vi "ImageRecon.vi"(7 "Logging queue element in":T1={"Imaging Protocol"=enum."Live Imaging", "Number of Trials"=0, "Frame Size"=512, "# Averaged frames"=0, "Dwell time (us)"=0.0, "Index of Z-plane"=0, "Timelapse?"=FALSE, "Logging process is active"=FALSE, "Speed logging enabled"=FALSE, "tdms file ref"=refnum, "path"=path "", "Trial Number"=0, "Expected # points acquired"=FALSE, "Manually stopped"=FALSE, "Last trial"=FALSE, "Ch0 data"=[], "Ch1 data"=[], "Image Time"=[], "Continuous Time"=[], "Points acquired"={"Ch0 last trial"=0, "Ch1 last trial"=0, "All trials"=0}, "HW Timings File"=refnum} {"Frame Size" items=["100X100"=100, "128X128"=128, "200X200"=200, "256X256"=256, "512X512"=512, "1024x1024"=1024, "2048x2048"=2048]; "Dwell time (us)" format="%#.6g"}, 8 "Error In":errorcluster, 9 "Data":T5, 10 "Frame Size":T3=200 items=["100X100"=100, "128X128"=128, "200X200"=200, "256X256"=256, "512X512"=512, "1024x1024"=1024, "2048x2048"=2048], 11 "Image Array (in)":T6) -> (0 "Error Out":errorcluster, 1 "Ch1-Green":i16[][](graph), 2 "Ch0-Red":i16[][](graph), 3 "Image Array(out)":T6)   [LabVIEW 2017]
uses:
  Typedefs/Frame Size.ctl
  Queue/Live graphs queue/Typedefs/Live imaging queue element.ctl
  <vilib>/vision/Image Controls.llb/IMAQ Image.ctl
  Typedefs/Frame data dual cluster.ctl
  Typedefs/Logging queue element.ctl
  Typedefs/Imaging Protocols enum.ctl
  Typedefs/Acquired points count.ctl
  Global Variables/gl_Images.vi
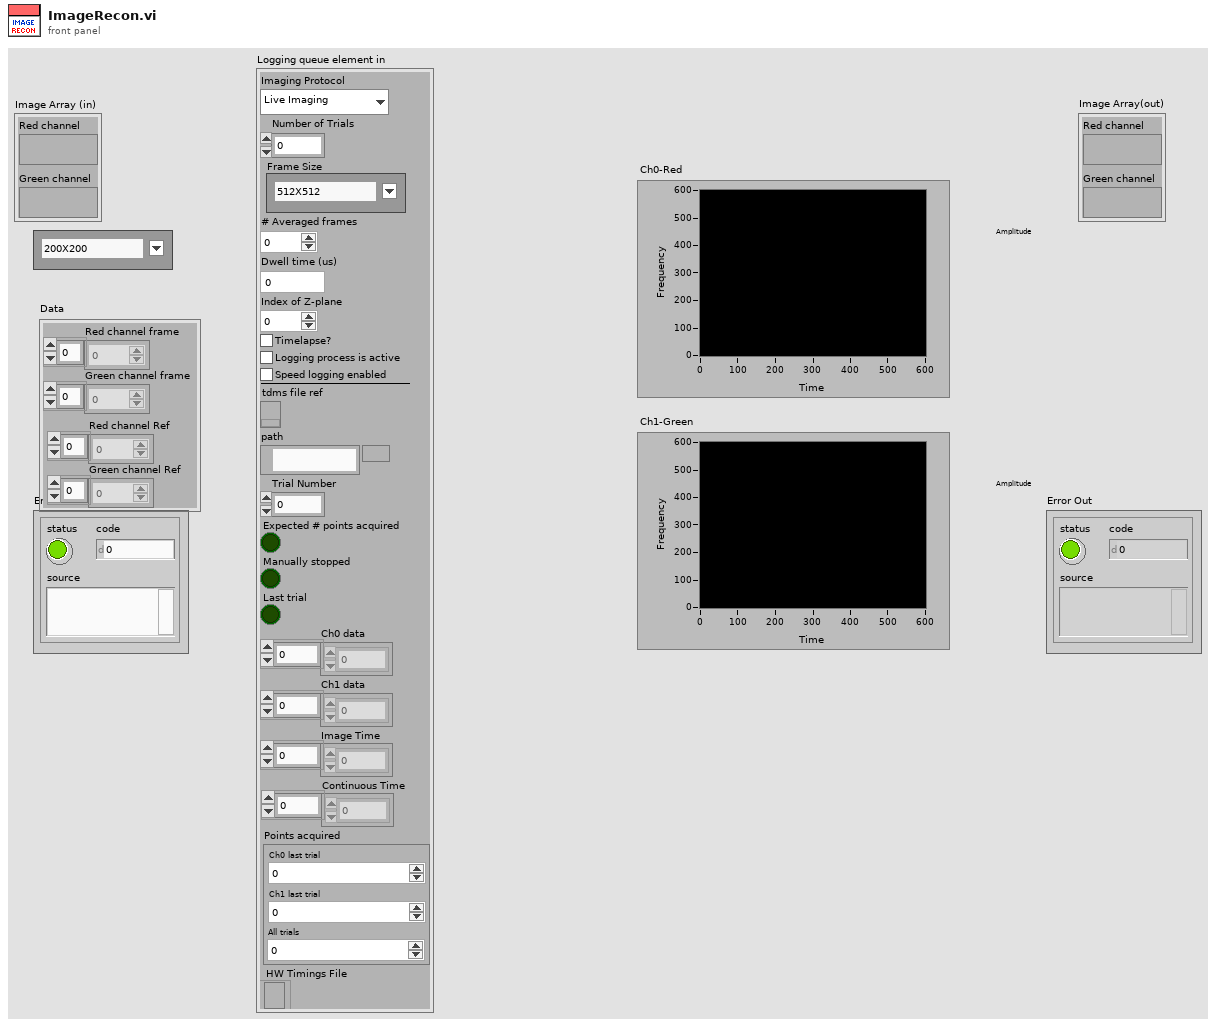
[diagram p1: front panel]
types:
  T1 = typedef "Logging queue element.ctl" = cluster{"Imaging Protocol":T2, "Number of Trials":u16, "Frame Size":T3, "# Averaged frames":u16, "Dwell time (us)":dbl, "Index of Z-plane":i32, "Timelapse?":bool, "Logging process is active":bool, "Speed logging enabled":bool, "tdms file ref":refnum<k34>, "path":path, "Trial Number":i32, "Expected # points acquired":bool, "Manually stopped":bool, "Last trial":bool, "Ch0 data":u32[], "Ch1 data":u32[], "Image Time":u64[], "Continuous Time":u64[], "Points acquired":T4, "HW Timings File":refnum<file>}
  T2 = typedef "Imaging Protocols enum.ctl" = enum16{"AOL Z-Stack", "Motor Z Stack", "Functional Acquisition", "Single Plane Acquisition", "Volume Acquisition", "Live Imaging", "Live Plane Imaging", "Live Volume Imaging"}
  T3 = typedef "Frame Size.ctl" = u16
  T4 = typedef "Acquired points count.ctl" = cluster{"Ch0 last trial":u64, "Ch1 last trial":u64, "All trials":u64}
  T5 = typedef "Frame data dual cluster.ctl" = cluster{"Red channel frame":dbl[], "Green channel frame":dbl[], "Red channel Ref":dbl[], "Green channel Ref":dbl[]}
  T6 = typedef "Live imaging queue element.ctl" = cluster{"Red channel":T7, "Green channel":T7}
  T7 = typedef "IMAQ Image.ctl" = refnum<image>
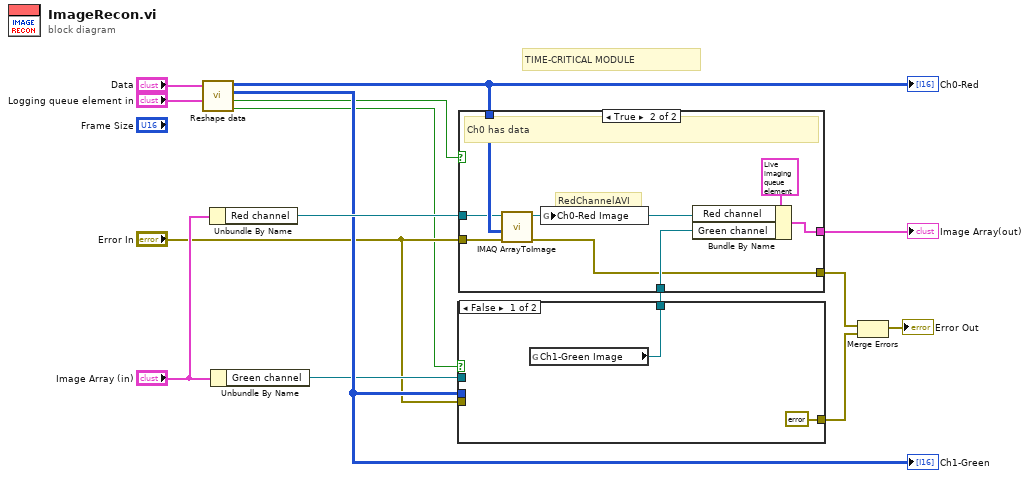
[diagram p0: block diagram]
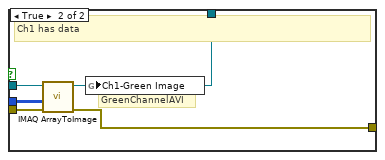
[diagram p2: hidden frame]
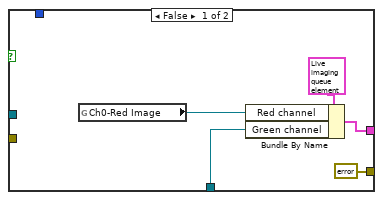
[diagram p3: hidden frame]
diagram:
  # "TIME-CRITICAL MODULE"
  n1 = call "Reshape data.vi"("Logging queue element in"="Logging queue element in", "Data"="Data") -> ("Ch1 has data"=w4:bool, "Ch0 has data"=w5:bool, "Ch1-Green"=w11:i16[][], "Ch0-Red"=w15:i16[][])  [unwired: 6 in]
  "Ch0-Red" <- w15
  "Ch1-Green" <- w11
  n2 = Unbundle By Name("Image Array (in)") -> ("Red channel"=w14:T7)
  n3 = Unbundle By Name("Image Array (in)") -> ("Green channel"=w10:T7)
  n4 = case shown="False" w4 {
    tunnel: w11 -> [_ w22]
    tunnel: w10 -> [_ w21]
    tunnel: "Error In" -> [_ w20]
    tunnel: [w17 w19] -> w6
    tunnel: [errorcluster {"status"=FALSE, "code"=0, "source"=""} ("error out") w18] -> w3
    frame False {
      n5 = global read "gl_Images.vi" "Ch1-Green Image"() -> (w17:T7)
    }
    frame True {
      # "GreenChannelAVI"
      # "Ch1 has data"
      n6 = call "IMAQ ArrayToImage"("error in (no error)"=w20, "Image Pixels (I16)"=w22, "Image"=w21) -> ("error out"=w18:errorcluster, "Image Out"=w19:T7)  [unwired: 7 in]
      n7 = global write "gl_Images.vi" "Ch1-Green Image"(w19) -> ()
    }
  }
  n8 = case shown="True" w5 {
    tunnel: w15 -> [_ w35]
    tunnel: w14 -> [_ w34]
    tunnel: [w25 w33] -> w13
    tunnel: "Error In" -> [_ w32]
    tunnel: w6 -> [w24 w30]
    tunnel: [errorcluster {"status"=FALSE, "code"=0, "source"=""} ("error out") w28] -> w2
    frame False {
      n9 = global read "gl_Images.vi" "Ch0-Red Image"() -> (w27:T7)
      n10 = Bundle By Name(cluster=T6 {"Red channel"=refnum, "Green channel"=refnum} ("Image Array(out)"), "Red channel"=w27, "Green channel"=w24) -> (w25:T6)
    }
    frame True {
      # "RedChannelAVI"
      # "Ch0 has data"
      n11 = call "IMAQ ArrayToImage"("error in (no error)"=w32, "Image Pixels (I16)"=w35, "Image"=w34) -> ("error out"=w28:errorcluster, "Image Out"=w31:T7)  [unwired: 7 in]
      n12 = global write "gl_Images.vi" "Ch0-Red Image"(w31) -> ()
      n13 = Bundle By Name(cluster=T6 {"Red channel"=refnum, "Green channel"=refnum} ("Image Array(out)"), "Red channel"=w31, "Green channel"=w30) -> (w33:T6)
    }
  }
  "Image Array(out)" <- w13
  n14 = Merge Errors(w2, w3) -> (→"Error Out":errorcluster)
